vi "Get Tasks.vi"(8 "error in (no error)":errorcluster, 10 "Project GID":string, 11 "Asana in":refnum<class "Asana.lvclass">) -> (0 "error out":errorcluster, 2 "Tasks Out":T1(array[cluster]), 3 "Asana out":refnum<class "Asana.lvclass">)   [LabVIEW 2016, in "Asana.lvclass"]
uses:
  Asana.lvclass
  Asana.lvclass/Asana.ctl
  <vilib>/addons/_JKI.lib/REST Client/classes/REST Client/REST Client.lvclass
  <vilib>/addons/_JKI.lib/Serialization/JSON/JKI JSON Serialization.lvlib
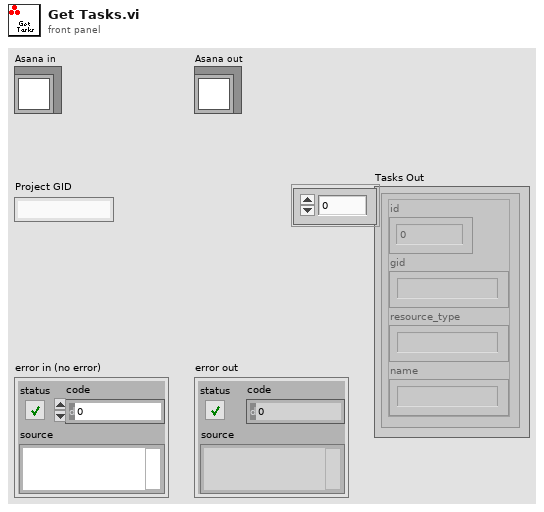
[diagram p1: front panel]
types:
  T1 = cluster{"id":i32, "gid":string, "resource_type":string, "name":string}[]
  T2 = cluster{"data":cluster{"id":i64, "gid":string, "resource_type":string, "name":string}[]}
  T3 = typedef "REST Client.lvlib/REST Client.lvclass/HTTP Header.ctl" = cluster{"header":string, "value":string}
  T4 = cluster{"id":i64, "gid":string, "resource_type":string, "name":string}[]
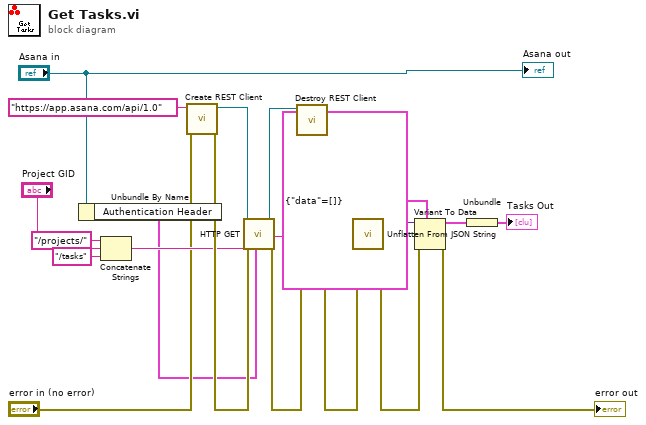
[diagram p0: block diagram]
diagram:
  w5 = T2 {"data"=[]}
  n1 = Unbundle By Name("Asana in") -> ("Authentication Header"=w2:T3[])
  n2 = Concatenate Strings("/projects/" ("string"), "Project GID", "/tasks" ("string")) -> (w15:string)
  n3 = call <vilib>:"Create REST Client.vi"("error in (no error)"="error in (no error)", "Base URL"="https://app.asana.com/api/1.0") -> ("error out"=w18:errorcluster, "REST Client out"=w20:refnum<class "REST Client.lvclass">)  [unwired: 8 in]
  n4 = call-dynamic "HTTP GET.vi"("request specific headers"=w2, "error in (no error)"=w18, "Path"=w15, "REST Client in"=w20) -> ("error out"=w10:errorcluster, "Response body"=w12:string, "REST Client out"=w19:refnum<class "REST Client.lvclass">)  [unwired: 2 in, 3 out]
  n5 = call-dynamic "Destroy REST Client.vi"("error in (no error)"=w10, "REST Client in"=w19) -> ("error out"=w9:errorcluster)  [unwired: 9 in]
  n6 = call <vilib>:"Unflatten From JSON String.vi"("Type and Defaults"=w5, "error in (no error)"=w9, "JSON String"=w12) -> ("error out"=w8:errorcluster, "Variant"=w11:variant)  [unwired: 7 in]
  n7 = Variant To Data(error in=w8, type=w5, Variant=w11) -> (data=w4:T2, error out=→"error out":errorcluster)
  n8 = Unbundle(w4) -> ("data"=→"Tasks Out":T4)
  "Asana out" <- "Asana in"
